vi "圆面积.vi"(11 "Radious":dbl) -> (3 "Area":dbl=nan)   [LabVIEW 2012]
doc: "功能：\n计算圆形面积。\n\n公式：\ns=Pi*r^2"
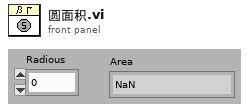
[diagram p1: front panel]
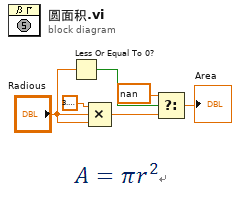
[diagram p0: block diagram]
diagram:
  n1 = Less Or Equal To 0?(x="Radious") -> (x <= 0?=w6:bool)
  n2 = Compound Arithmetic op=MULTIPLY(3.141592653589793, "Radious", "Radious") -> (w2:dbl)
  n3 = Select(t=nan, s=w6, f=w2) -> (s? t:f=→"Area":dbl)
